vi "Copy Pixmap to Image (ARGB with Mask Output).vi"(8 "error in (no error)":errorcluster, 9 "Greyscale Image Mask Destination in":T1, 10 "ARGB Image Destination in":T3, 11 "Pixmap Image Data":T2) -> (0 "error out":errorcluster, 2 "Greyscale Image Mask Destination":T1, 3 "ARGB Image Destination":T3)   [LabVIEW 2020, in "image.lvlib"]
doc: "Copy the Flattened Pixmap Image Data to the Image Destination. The Image Destination will be resized to fit the Pixmap Image Data. If the Pixmap Image Data contains mask information then the mask will be converted to a Greyscale Mask. The Greyscale Mask destination will also be resized to fit the mask data.\n\nOnly 8, 24 or 32 bit Pixmap types are supported."
uses:
  image.lvlib
  ARGB Image.ctl
  Greyscale Image.ctl
  <vilib>/picture/picture.llb/imagedata.ctl
  a116197e-b340-4968-94fb-08de404a21d3.vi
  FixPixmap.vi
  Default8bitColourMap.vi
  <vilib>/Utility/error.llb/Error Cluster From Error Code.vi
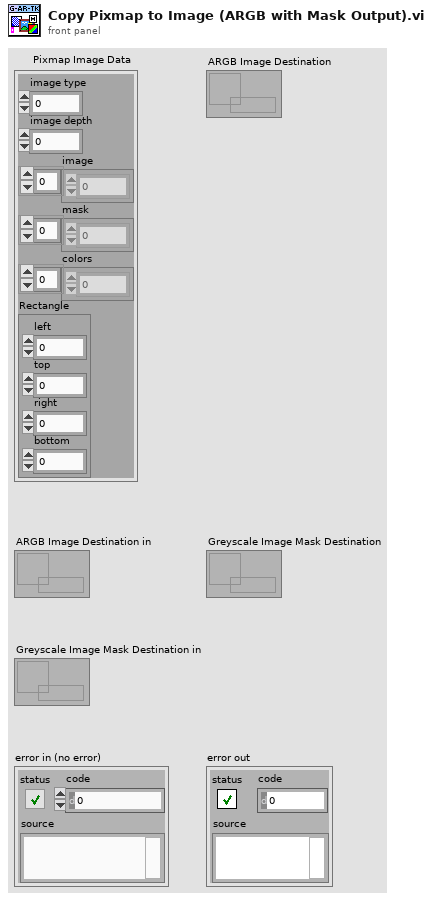
[diagram p1: front panel]
types:
  T1 = typedef "image.lvlib/Greyscale Image.ctl" = refnum<data-value>
  T2 = typedef "imagedata.ctl" = cluster{"image type":i32, "image depth":i32, "image":u8[], "mask":u8[], "colors":u32[], "Rectangle":cluster{"left":i16, "top":i16, "right":i16, "bottom":i16}}
  T3 = typedef "image.lvlib/ARGB Image.ctl" = refnum<data-value>
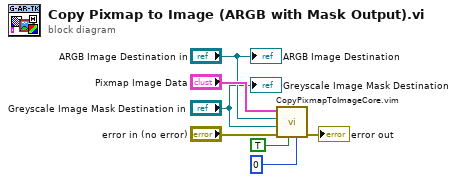
[diagram p0: block diagram]
diagram:
  n1 = call "CopyPixmapToImageCore.vim"("Background Value"=u32 0, "Has Mask"=TRUE, "error in (no error)"="error in (no error)", "Mask Image"="Greyscale Image Mask Destination in", "Source Image"="ARGB Image Destination in", "image data"="Pixmap Image Data") -> ("error out"=→"error out":errorcluster)  [unwired: 5 in]
  "ARGB Image Destination" <- "ARGB Image Destination in"
  "Greyscale Image Mask Destination" <- "Greyscale Image Mask Destination in"
